vi "SwissSPAD Live_Correct SS3 Gate Slippage [U8].vi"(8 "Error In":errorcluster, 9 "Slippage Correction (T)":bool=TRUE, 11 "Array in":u8[][](array[numeric])) -> (0 "Error Out":errorcluster, 2 "Last Strip Saturated?":bool, 3 "Array out":u8[][](array[numeric]))   [LabVIEW 2021]
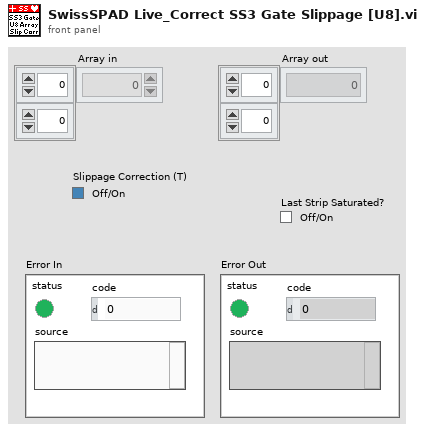
[diagram p1: front panel]
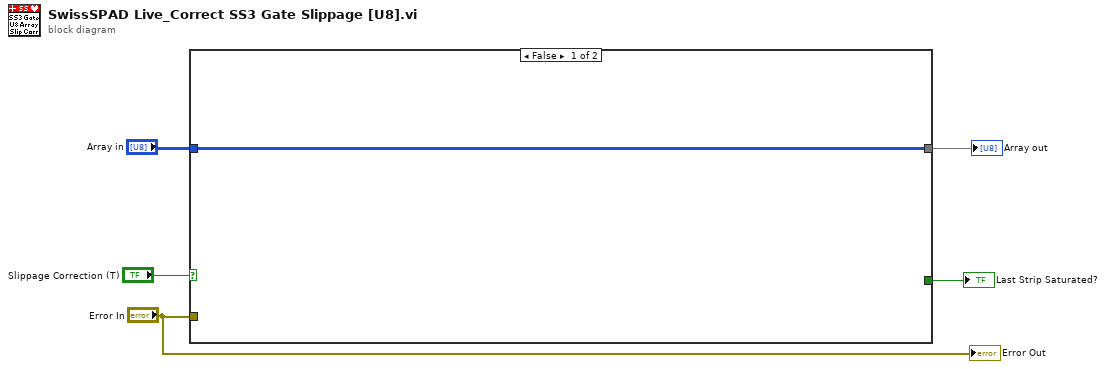
[diagram p0: block diagram]
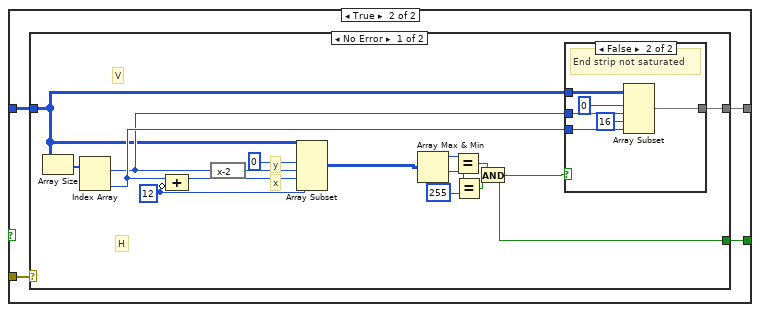
[diagram p2: hidden frame]
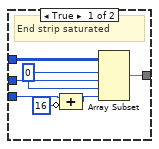
[diagram p3: hidden frame]
diagram:
  n1 = case shown="False" "Slippage Correction (T)" {
    tunnel: [_ w10] -> w5
    tunnel: [w6 w9] -> w4
    tunnel: "Array in" -> [w6 w8]
    tunnel: "Error In" -> [_ w7]
    frame False {
    }
    frame True {
      n2 = case shown="No Error" w7 {
        tunnel: [w22 _] -> w10
        tunnel: [w20 w40] -> w9
        tunnel: w8 -> [w18 w40]
        frame No Error {
          w21 = 12 ("value")
          # "H"
          # "V"
          # "x"
          # "y"
          n3 = Array Size(array=w18) -> (size(s)=w11:i32[])
          n4 = Index Array(array=w11) -> (element #1=w23:i32, element #2=w24:i32)  [unwired: 2 in]
          n5 = Compound Arithmetic op=ADD(w24, invert w21) -> (w19:i32)
          n6 = expression code="x-2"(w23) -> (w26:i32)
          n7 = Array Subset(array=w18, index (row)=0 ("length"), length (row)=w26, index (col)=w19, length (col)=w21) -> (w25:u8[][])
          n8 = Array Max & Min(array=w25) -> (max value=w13:u8, min value=w14:u8)  [unwired: 2 out]
          n9 = Equal?(x=w13, y=w14) -> (x = y?=w16:bool)
          n10 = Equal?(x=w14, y=u8 255) -> (x = y?=w17:bool)
          n11 = And(x=w16, y=w17) -> (x .and. y?=w22:bool)
          n12 = case shown="False" w22 {
            tunnel: w18 -> [w33 w39]
            tunnel: w23 -> [w32 w38]
            tunnel: w24 -> [w28 w36]
            tunnel: [w30 w35] -> w20
            frame True {
              w31 = 0 ("index")
              # "End strip saturated"
              n13 = Compound Arithmetic op=ADD(w28, invert 16 ("value")) -> (w27:i32)
              n14 = Array Subset(array=w33, index (row)=w31, length (row)=w32, index (col)=w31, length (col)=w27) -> (w30:u8[][])
            }
            frame False {
              # "End strip not saturated"
              n15 = Array Subset(array=w39, index (row)=0 ("index"), length (row)=w38, index (col)=16 ("index"), length (col)=w36) -> (w35:u8[][])
            }
          }
        }
        frame Error {
        }
      }
    }
  }
  "Last Strip Saturated?" <- w5
  "Array out" <- w4
  "Error Out" <- "Error In"
